vi "Initialize Coin.vi"(8 "error in (no error)":errorcluster, 11 "Monedas in":refnum<class "Monedas.lvclass">) -> (0 "error out":errorcluster, 3 "Monedas out":refnum<class "Monedas.lvclass">)   [LabVIEW 2020, in "Monedas.lvlib" / "Monedas.lvclass"]
uses:
  Monedas.lvclass
  Monedas.lvclass/Monedas.ctl
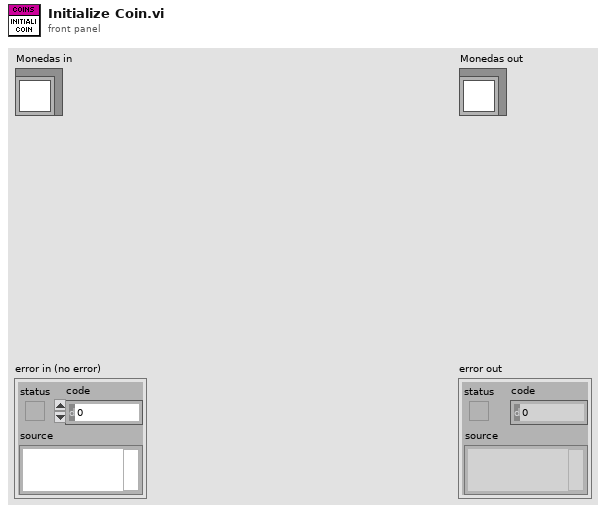
[diagram p1: front panel]
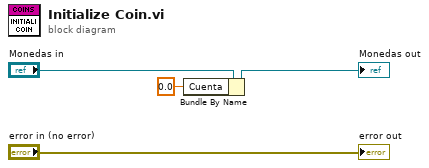
[diagram p0: block diagram]
diagram:
  n1 = Bundle By Name(cluster="Monedas in", "Cuenta"=0.0) -> (→"Monedas out":refnum<class "Monedas.lvclass">)
  "error out" <- "error in (no error)"
